vi "ButtonResetBarrelGrabbers.vi"(11 "Buttons":bool[](array[boolean])) -> ()   [LabVIEW 2014]
uses:
  <vilib>/Rock Robotics/WPI/CAN/TalonSRX/WPI_CANTalonSRX_APIFeedbackSelect.ctl
  <vilib>/Rock Robotics/WPI/CAN/TalonSRX/WPI_CANTalonSRX_APIControlMode.ctl
  Utilities/CanGrabberSetpoint.vi
panel:
  out "Encoder Velocity 2":dbl
  in  "Arm PID Gains":T1={"proportional gain (Kc)"=10.0, "integral time (Ti, min)"=0.0, "derivative time (Td, min)"=2.0}
  out "Encoder Velocity":dbl
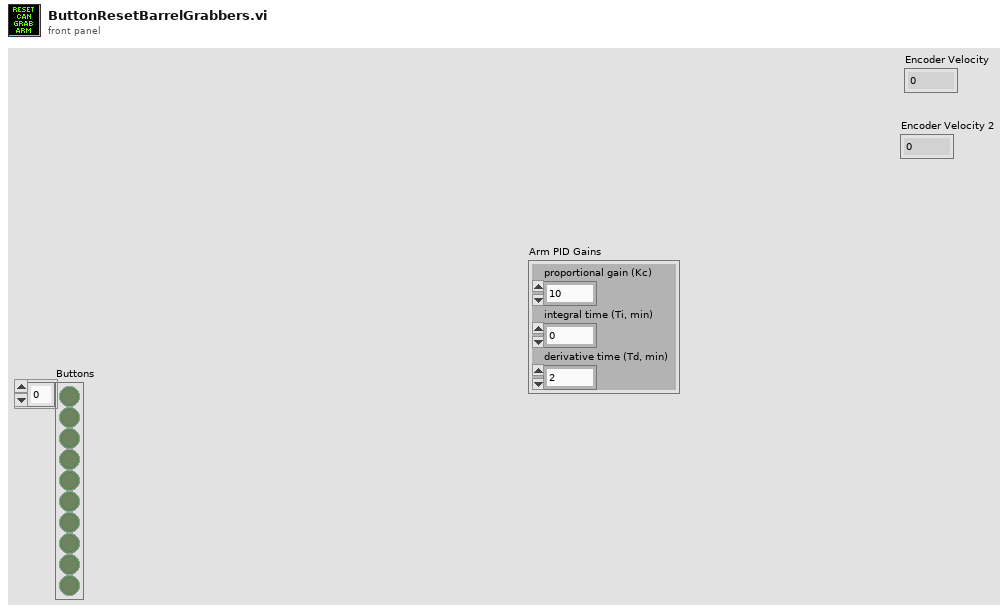
[diagram p1: front panel]
types:
  T1 = cluster{"proportional gain (Kc)":dbl, "integral time (Ti, min)":dbl, "derivative time (Td, min)":dbl}
  T2 = typedef "WPI_CANTalonSRX_APIControlMode.ctl" = enum8{"Percent VBus", "Speed", "Position", "Slave", "Unchanged / Invalid"}
  T3 = typedef "WPI_CANTalonSRX_APIFeedbackSelect.ctl" = enum16{"Digital Quadrature Encoder", "Analog Potentiometer", "Analog Encoder"}
  T4 = typedef "WPI_MotorControlDeviceRef.ctl" = cluster{"DeviceStatus":errorcluster, "Type":T5, "PWM":cluster{"Controller":T6, "PWM Channel":T7, "DeadBand":T8}, "CAN":cluster{"Device Number":u8, "Control Mode":T9, "Semaphore":T10, "Max Vout":dbl, "TalonSRX Control Mode":T2}, "Invert":bool, "TransformRef":T11, "InvTransformRef":T11}
  T5 = typedef "WPI_MotorControlType.ctl" = enum16{"PWM", "CAN", "CANTalonSRX"}
  T6 = typedef "FPGA_TypedefDigitalModule.ctl" = enum16{"Controller 1"}
  T7 = typedef "FPGA_DIOPWMChannel.ctl" = enum8{"PWM 0", "PWM 1", "PWM 2", "PWM 3", "PWM 4", "PWM 5", "PWM 6", "PWM 7", "PWM 8", "PWM 9", "PWM MXP 0", "PWM MXP 1", "PWM MXP 2", "PWM MXP 3", "PWM MXP 4", "PWM MXP 5", "PWM MXP 6", "PWM MXP 7", "PWM MXP 8", "PWM MXP 9", "Invalid"}
  T8 = typedef "WPI_PWMDeadband.ctl" = cluster{"Name":string, "maxPositivePwm":i32, "minPositivePwm":i32, "centerPwm":i32, "maxNegativePwm":i32, "minNegativePwm":i32, "angularRange":u16}
  T9 = typedef "WPI_CANJaguar_ControlMode.ctl" = enum8{"Percent VBus", "Current", "Speed", "Position", "Voltage"}
  T10 = typedef "Semaphore RefNum" = refnum<k1>
  T11 = typedef "WPI_PWMTransform_ConPane.ctl" = refnum<vi>
  T12 = typedef "WPI_CANTalonSRX_GlobalStatus.ctl" = cluster{"Applied Throttle":dbl, "Module Enabled":bool, "CAN Error":errorcluster, "Closed Loop Error":dbl, "Forward Limit Switch Closed":bool, "Reverse Limit Switch Closed":bool, "Sensor Position":dbl, "Sensor Velocity":dbl, "Current":dbl, "Sticky Fault - Over Temp":bool, "Sticky Fault - Under Voltage":bool, "Sticky Fault - Forward Limit":bool, "Sticky Fault - Reverse Limit":bool, "Sticky Fault - Forward Soft Limit":bool, "Sticky Fault - Reverse Soft Limit":bool, "Brake is Enabled":bool, "Encoder Position":dbl, "Encoder Velocity":dbl, "Encoder Index Count":dbl, "Encoder A Pin State":bool, "Encoder B Pin State":bool, "Encoder Index Pin State":bool, "Analog In":dbl, "Analog In Velocity":dbl, "Temperature (C)":dbl, "Battery Voltage":dbl}
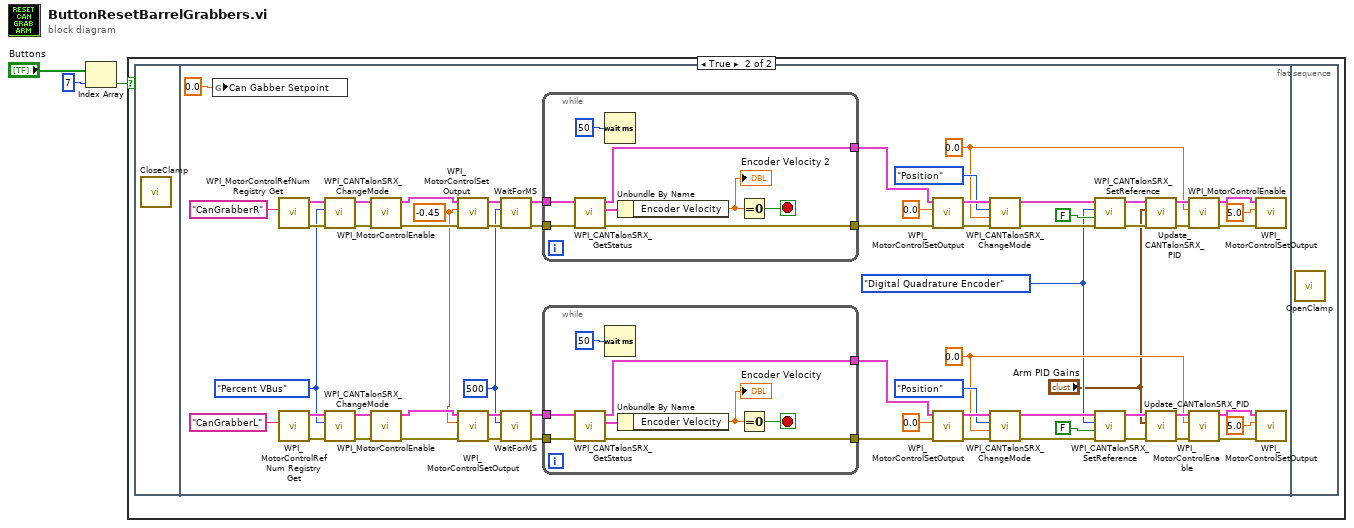
[diagram p0: block diagram]
diagram:
  n1 = Index Array(array="Buttons", index=7) -> (element=w1:bool)
  n2 = case shown="True" w1 {
    frame False {
    }
    frame True {
      n3 = flat-sequence {
        frame #0 {
          n4 = call "CloseClamp.vi"() -> ()  [unwired: 12 in]
        }
        frame #1 {
          w5 = u32 500 ("milliseconds to wait")
          w26 = 0.0 ("Output")
          w4 = -0.45 ("Output")
          w21 = WPI_CANTalonSRX_APIControlMode."Percent VBus" ("Control Mode")
          w23 = WPI_CANTalonSRX_APIFeedbackSelect."Digital Quadrature Encoder" ("Feedback Reference")
          w47 = 0.0 ("Output")
          n5 = global write "CanGrabberSetpoint.vi" "Can Gabber Setpoint"(0.0 ("Can Gabber Setpoint")) -> ()
          n6 = call <vilib>:"WPI_MotorControlRefNum Registry Get.vi"("refnum name"="CanGrabberR") -> ("error out"=w24:errorcluster, "MotorControlDevRef"=w25:T4)  [unwired: 9 in]
          n7 = call <vilib>:"WPI_MotorControlRefNum Registry Get.vi"("refnum name"="CanGrabberL") -> ("error out"=w45:errorcluster, "MotorControlDevRef"=w46:T4)  [unwired: 9 in]
          n8 = call <vilib>:"WPI_CANTalonSRX_ChangeMode.vi"("error in (no error)"=w24, "Control Mode"=w21, "CAN Talon SRX Ref"=w25) -> ("error out"=w14:errorcluster, "CAN Talon SRX Ref Out"=w13:T4)  [unwired: 7 in]
          n9 = call <vilib>:"WPI_CANTalonSRX_ChangeMode.vi"("error in (no error)"=w45, "Control Mode"=w21, "CAN Talon SRX Ref"=w46) -> ("error out"=w9:errorcluster, "CAN Talon SRX Ref Out"=w10:T4)  [unwired: 7 in]
          n10 = call <vilib>:"WPI_MotorControlEnable.vi"("error in (no error)"=w14, "CAN Jaguar Ref"=w13) -> ("error out"=w11:errorcluster, "CAN Jaguar Ref Out"=w12:T4)  [unwired: 8 in]
          n11 = call <vilib>:"WPI_MotorControlEnable.vi"("error in (no error)"=w9, "CAN Jaguar Ref"=w10) -> ("error out"=w7:errorcluster, "CAN Jaguar Ref Out"=w8:T4)  [unwired: 8 in]
          n12 = call <vilib>:"WPI_MotorControlSetOutput.vi"("error in (no error)"=w11, "Output"=w4, "MotorControlDevRef"=w12) -> ("error out"=w37:errorcluster, "MotorControlDevRef"=w38:T4)  [unwired: 6 in, 1 out]
          n13 = call <vilib>:"WPI_MotorControlSetOutput.vi"("error in (no error)"=w7, "Output"=w4, "MotorControlDevRef"=w8) -> ("error out"=w58:errorcluster, "MotorControlDevRef"=w59:T4)  [unwired: 6 in, 1 out]
          n14 = call "WaitForMS.vi"("error in"=w37, "milliseconds to wait"=w5, "MotorControlDevRef"=w38) -> ("error out"=w35:errorcluster, "MotorControlDevRef 2"=w36:T4)  [unwired: 7 in]
          n15 = call "WaitForMS.vi"("error in"=w58, "milliseconds to wait"=w5, "MotorControlDevRef"=w59) -> ("error out"=w56:errorcluster, "MotorControlDevRef 2"=w57:T4)  [unwired: 7 in]
          n16 = while {
            tunnel: w36 -> [w72]
            tunnel: w35 -> [w71]
            tunnel: [w68] -> w40
            tunnel: [w67] -> w39
            stop <- w66 stop-if-true
            n17 = call <vilib>:"WPI_CANTalonSRX_GetStatus.vi"("error in (no error)"=w71, "CAN Talon SRX Ref"=w72) -> ("error out"=w67:errorcluster, "Talon SRX Status"=w70:T12, "CAN Talon SRX Ref Out"=w68:T4)  [unwired: 7 in]
            n18 = Wait (ms)(milliseconds to wait=u32 50) -> ()  [unwired: 1 out]
            n19 = Unbundle By Name(w70) -> ("Encoder Velocity"=w69:dbl)
            "Encoder Velocity 2" <- w69
            n20 = Equal To 0?(x=w69) -> (x = 0?=w66:bool)
          }
          n21 = while {
            tunnel: w57 -> [w80]
            tunnel: w56 -> [w79]
            tunnel: [w76] -> w61
            tunnel: [w75] -> w60
            stop <- w74 stop-if-true
            n22 = call <vilib>:"WPI_CANTalonSRX_GetStatus.vi"("error in (no error)"=w79, "CAN Talon SRX Ref"=w80) -> ("error out"=w75:errorcluster, "Talon SRX Status"=w78:T12, "CAN Talon SRX Ref Out"=w76:T4)  [unwired: 7 in]
            n23 = Wait (ms)(milliseconds to wait=u32 50) -> ()  [unwired: 1 out]
            n24 = Unbundle By Name(w78) -> ("Encoder Velocity"=w77:dbl)
            "Encoder Velocity" <- w77
            n25 = Equal To 0?(x=w77) -> (x = 0?=w74:bool)
          }
          n26 = call <vilib>:"WPI_MotorControlSetOutput.vi"("error in (no error)"=w39, "Output"=0.0, "MotorControlDevRef"=w40) -> ("error out"=w41:errorcluster, "MotorControlDevRef"=w42:T4)  [unwired: 6 in, 1 out]
          n27 = call <vilib>:"WPI_MotorControlSetOutput.vi"("error in (no error)"=w60, "Output"=0.0, "MotorControlDevRef"=w61) -> ("error out"=w62:errorcluster, "MotorControlDevRef"=w63:T4)  [unwired: 6 in, 1 out]
          n28 = call <vilib>:"WPI_CANTalonSRX_ChangeMode.vi"("error in (no error)"=w41, "Output"=w26, "Control Mode"=WPI_CANTalonSRX_APIControlMode."Position", "CAN Talon SRX Ref"=w42) -> ("error out"=w31:errorcluster, "CAN Talon SRX Ref Out"=w30:T4)  [unwired: 6 in]
          n29 = call <vilib>:"WPI_CANTalonSRX_ChangeMode.vi"("error in (no error)"=w62, "Output"=w47, "Control Mode"=WPI_CANTalonSRX_APIControlMode."Position", "CAN Talon SRX Ref"=w63) -> ("error out"=w52:errorcluster, "CAN Talon SRX Ref Out"=w51:T4)  [unwired: 6 in]
          n30 = call <vilib>:"WPI_CANTalonSRX_SetReference.vi"("error in (no error)"=w31, "Reverse Feedback Sensor"=FALSE, "Feedback Reference"=w23, "CAN Talon SRX Ref"=w30) -> ("error out"=w28:errorcluster, "CAN Talon SRX Ref Out"=w29:T4)  [unwired: 6 in]
          n31 = call <vilib>:"WPI_CANTalonSRX_SetReference.vi"("error in (no error)"=w52, "Reverse Feedback Sensor"=FALSE, "Feedback Reference"=w23, "CAN Talon SRX Ref"=w51) -> ("error out"=w49:errorcluster, "CAN Talon SRX Ref Out"=w50:T4)  [unwired: 6 in]
          n32 = call "Update_CANTalonSRX_PID.vi"("error in (no error)"=w28, "PID Gains"="Arm PID Gains", "CAN Talon SRX Ref"=w29) -> ("error out"=w32:errorcluster, "CAN Talon SRX Ref Out"=w33:T4)  [unwired: 7 in]
          n33 = call "Update_CANTalonSRX_PID.vi"("error in (no error)"=w49, "PID Gains"="Arm PID Gains", "CAN Talon SRX Ref"=w50) -> ("error out"=w53:errorcluster, "CAN Talon SRX Ref Out"=w54:T4)  [unwired: 7 in]
          n34 = call <vilib>:"WPI_MotorControlEnable.vi"("error in (no error)"=w32, "Encoder Initial Position"=w26, "CAN Jaguar Ref"=w33) -> ("error out"=w20:errorcluster, "CAN Jaguar Ref Out"=w19:T4)  [unwired: 7 in]
          n35 = call <vilib>:"WPI_MotorControlEnable.vi"("error in (no error)"=w53, "Encoder Initial Position"=w47, "CAN Jaguar Ref"=w54) -> ("error out"=w16:errorcluster, "CAN Jaguar Ref Out"=w17:T4)  [unwired: 7 in]
          n36 = call <vilib>:"WPI_MotorControlSetOutput.vi"("error in (no error)"=w20, "Output"=5.0, "MotorControlDevRef"=w19) -> ()  [unwired: 6 in, 3 out]
          n37 = call <vilib>:"WPI_MotorControlSetOutput.vi"("error in (no error)"=w16, "Output"=5.0, "MotorControlDevRef"=w17) -> ()  [unwired: 6 in, 3 out]
        }
        frame #2 {
          n38 = call "OpenClamp.vi"() -> ()  [unwired: 12 in]
        }
      }
    }
  }
